vi "Write Position.vi"(8 "error in (no error)":errorcluster, 10 "Position":T1, 11 "window in":refnum<class "window.lvclass">) -> (0 "error out":errorcluster, 3 "window out":refnum<class "window.lvclass">)   [LabVIEW 2013, in "frontPanelObjects.lvlib" / "window.lvclass"]
uses:
  window.lvclass
  <vilib>/Utility/miscctls.llb/LVPositionTypeDef.ctl
  window.lvclass/window.ctl
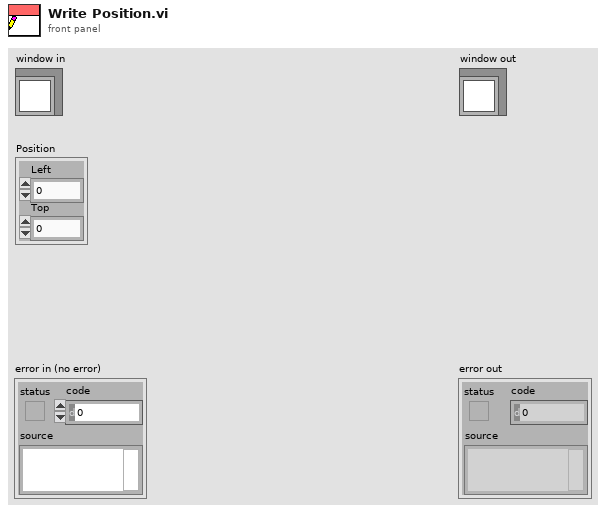
[diagram p1: front panel]
types:
  T1 = typedef "LVPositionTypeDef.ctl" = cluster{"Left":i32, "Top":i32}
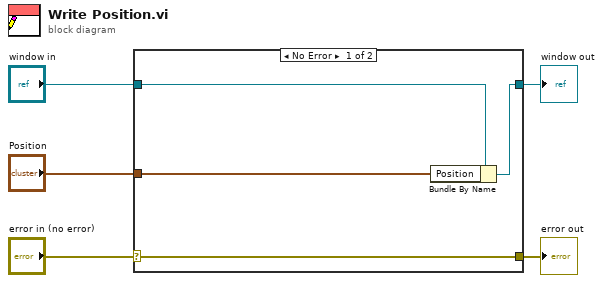
[diagram p0: block diagram]
diagram:
  n1 = case shown="No Error" "error in (no error)" {
    selector: "error in (no error)" -> [w9 w10]
    tunnel: [w9 w10] -> w4
    tunnel: [w7 w11] -> w2
    tunnel: "window in" -> [w8 w11]
    tunnel: "Position" -> [w6 _]
    frame No Error {
      n2 = Bundle By Name(cluster=w8, "Position"=w6) -> (w7:refnum<class "window.lvclass">)
    }
    frame Error {
    }
  }
  "error out" <- w4
  "window out" <- w2
